vi "Close XML.vi"(8 "error in (no error)":errorcluster, 11 "XML Handler in":refnum<class "XML Handler.lvclass">) -> (0 "error out":errorcluster, 3 "XML Handler out":refnum<class "XML Handler.lvclass">)   [LabVIEW 2020, in "XML Handler.lvclass"]
uses:
  XML Handler.lvclass
  XML Handler.lvclass/XML Handler.ctl
  <vilib>/xml/Close Reference(Node).vi
  <vilib>/xml/NI_XML.lvlib
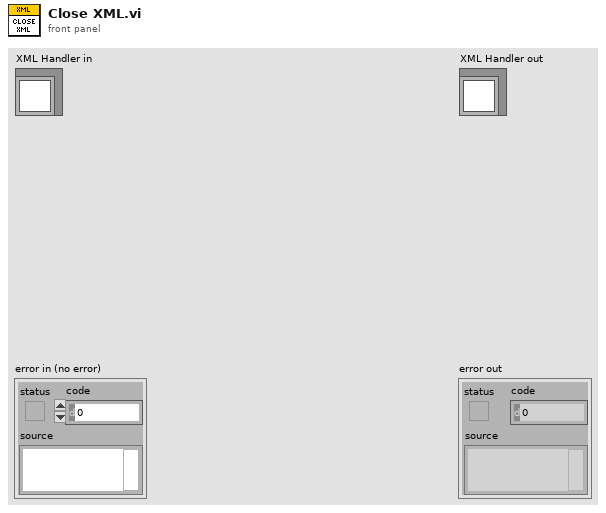
[diagram p1: front panel]
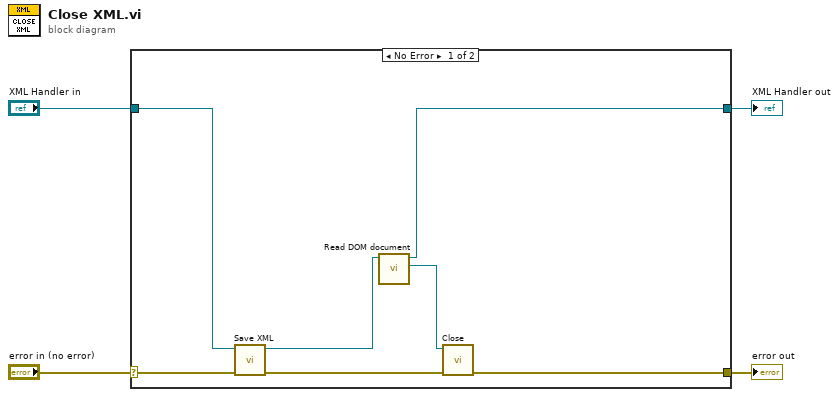
[diagram p0: block diagram]
diagram:
  n1 = case shown="No Error" "error in (no error)" {
    selector: "error in (no error)" -> [w10 w13]
    tunnel: [w6 w13] -> w3
    tunnel: [w5 w12] -> w1
    tunnel: "XML Handler in" -> [w11 w12]
    frame No Error {
      n2 = call "Save XML.vi"("error in (no error)"=w10, "XML Handler in"=w11) -> ("error out"=w7:errorcluster, "XML Handler out"=w9:refnum<class "XML Handler.lvclass">)  [unwired: 8 in]
      n3 = call "Read DOM document.vi"("XML Handler in"=w9) -> ("DOM document"=w8:refnum<k20>, "XML Handler out"=w5:refnum<class "XML Handler.lvclass">)  [unwired: 9 in]
      n4 = call-poly <vilib>:"Close.vi"("error in (no error)"=w7, "node"=w8) -> ("error out"=w6:errorcluster)  [unwired: 7 in]
    }
    frame Error {
    }
  }
  "error out" <- w3
  "XML Handler out" <- w1
